vi "VISA_ReadAndSave_2CHparalelos.vi"() -> ()   [LabVIEW 2019]
uses:
  813f916b-c519-439e-9418-14bd48b6d342.vi
  <vilib>/Instr/_visa.llb/VISA Configure Serial Port (Instr).vi
  <vilib>/Analysis/Matrix/Comparison/Not Equal/Not Equal.vi
  <vilib>/Analysis/Matrix/Comparison/Not Equal/Not Equal - RM,RM.vi
panel:
  out "error file":errorcluster
  in  "file name":string
  out "Plot 1":dbl[](graph)
  out "Plot 0":dbl[](graph)
  out "Status Read":errorcluster
  out "Buffer Array":dbl[](array[numeric])
  out "Read Buffer":string
  out "Status Serial":errorcluster
  in  "Stop Read":bool
  in  "Start Read":bool
  in  "baud rate (9600)":u32=115200
  in  "data bits (8)":u8=8 min=5 max=8 step=1
  in  "VISA resource name":refnum<visa-resource-name>
  # "Controle de Salvamento"
  # "Log de Erros"
  # "Conversão Para Inteiro"
  # "Resultado da Leitura"
  # "Controle da porta Serial USB"
  # "Controle da Leitura"
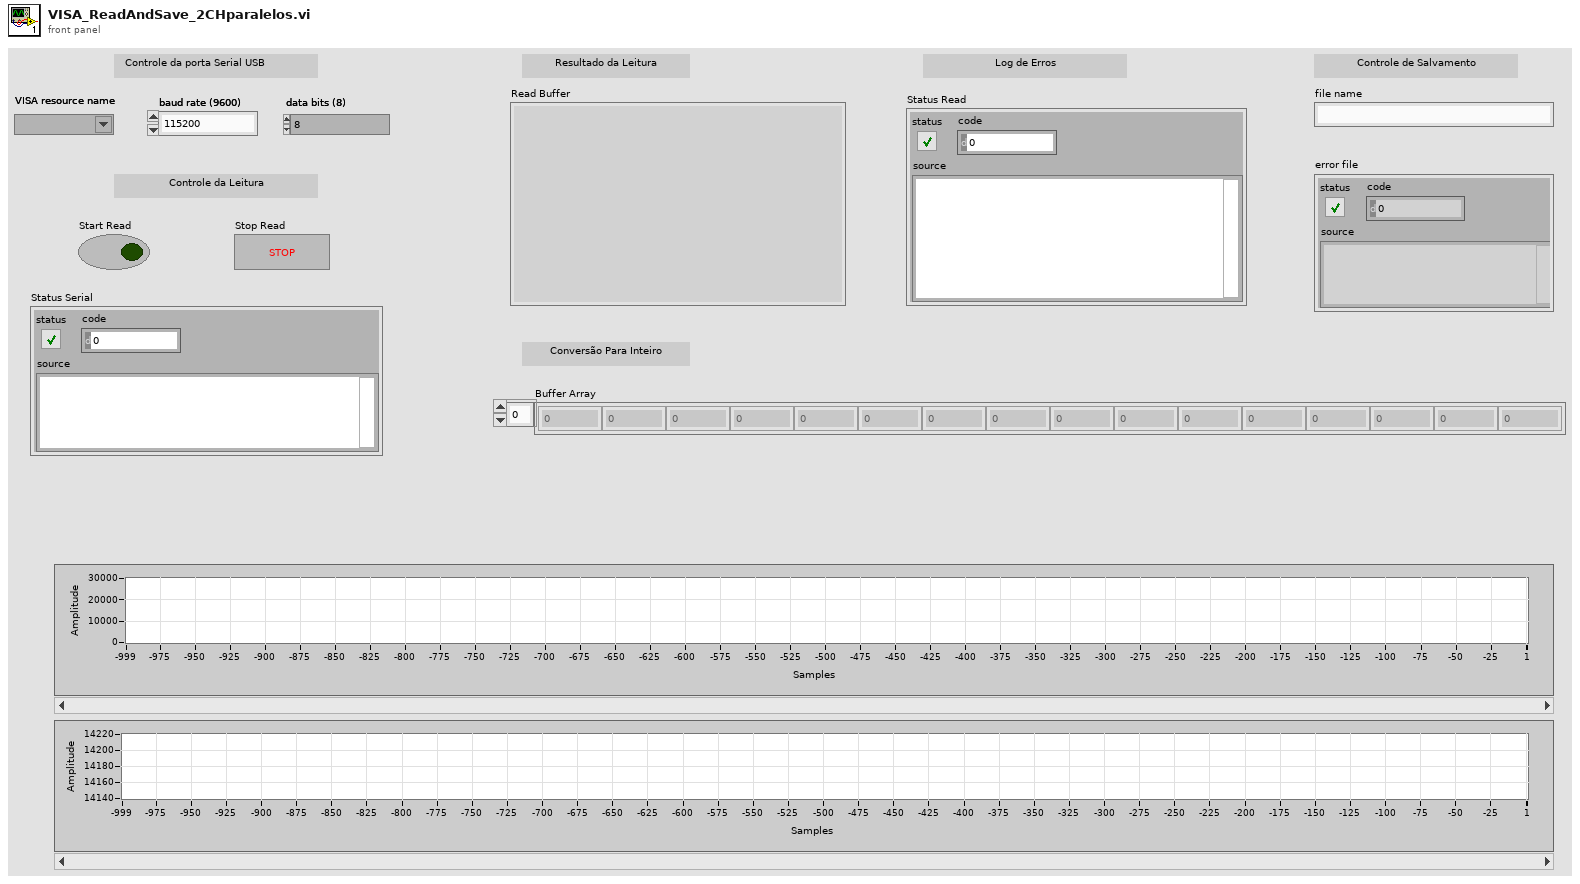
[diagram p1: front panel]
types:
  T1 = typedef "NI_Matrix.lvlib/RealMatrix.ctl" = dbl[][]
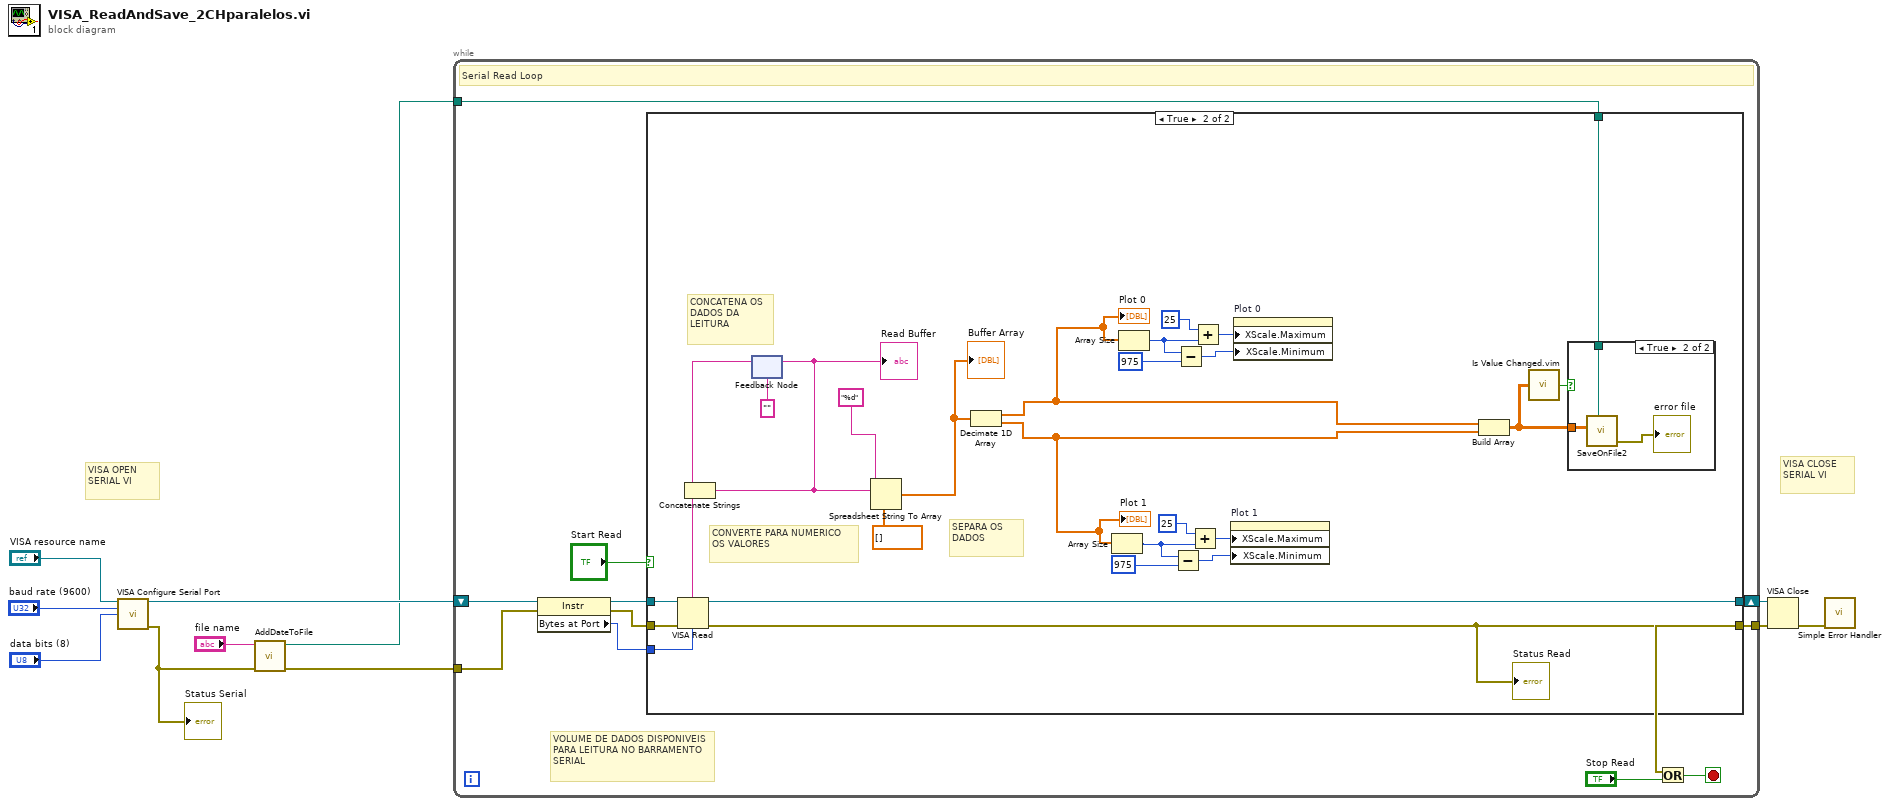
[diagram p0: block diagram]
diagram:
  # "VISA OPEN SERIAL VI"
  # "VISA CLOSE SERIAL VI"
  n1 = call-poly "VISA Configure Serial Port"("VISA resource name"="VISA resource name", "baud rate (9600)"="baud rate (9600)", "data bits (8)"="data bits (8)") -> ("VISA resource name out"=w9:refnum<visa-resource-name>, "error out"=w2:errorcluster)  [unwired: 11 in]
  "Status Serial" <- w2
  n2 = call "AddDateToFile.vi"("error in (no error)"=w2, "file name"="file name") -> ("error out"=w3:errorcluster, "new file path (Not A Path if cancelled)"=w1:path)  [unwired: 8 in]
  n3 = while {
    tunnel: w3 -> [w13]
    tunnel: [w20] -> w10
    shift-right: [w19] -> w8
    shift-left: w9 -> [w17]
    tunnel: w1 -> [w12]
    stop <- w18 stop-if-true
    # "VOLUME DE DADOS DISPONIVEIS PARA LEITURA NO BARRAMENTO SERIAL"
    # "Serial Read Loop"
    n4 = property class="Instr"(reference=w17, error in=w13) -> (reference out=w14:refnum<visa-resource-name>, error out=w15:errorcluster, "Bytes at Port"=w16:u32)
    n5 = case shown="True" "Start Read" {
      tunnel: [w23 w51] -> w20
      tunnel: [w24 w49] -> w19
      tunnel: w16 -> [_ w45]
      tunnel: w14 -> [w24 w44]
      tunnel: w15 -> [w23 w43]
      tunnel: w12 -> [_ w31]
      frame False {
        # "OS DADOS SÃO ACUMULADOS NO BUFFER ESPERANDO A PERMISSÃO PARA SER LIDOS"
      }
      frame True {
        # "SEPARA OS DADOS"
        # "CONVERTE PARA NUMERICO OS VALORES"
        # "CONCATENA OS DADOS DA LEITURA"
        n6 = VISA Read(VISA resource name=w44, byte count=w45, error in (no error)=w43) -> (VISA resource name out=w49:refnum<visa-resource-name>, read buffer=w40:string, error out=w51:errorcluster)  [unwired: 1 out]
        "Status Read" <- w51
        n7 = feedback #1("") -> (w46:string)
        n8 = Concatenate Strings(w46, w40) -> (w48:string)
        "Read Buffer" <- w48
        n9 = feedback-in #1(w48) -> ()
        n10 = Spreadsheet String To Array(format string="%d", spreadsheet string=w48, array type (2D Dbl)=dbl[] []) -> (array=w41:dbl[])  [unwired: 1 in]
        "Buffer Array" <- w41
        n11 = Decimate 1D Array(w41) -> (w32:dbl[], w25:dbl[])
        "Plot 0" <- w32
        "Plot 1" <- w25
        n12 = Array Size(array=w25) -> (size(s)=w27:i32)
        n13 = Array Size(array=w32) -> (size(s)=w35:i32)
        n14 = Subtract(x=w27, y=975) -> (x-y=w30:i32)
        n15 = Subtract(x=w35, y=975) -> (x-y=w36:i32)
        n16 = Add(x=25, y=w27) -> (x+y=w29:i32)
        n17 = Add(x=25, y=w35) -> (x+y=w34:i32)
        n18 = property on="Plot 1" class="WFGraph (strict)"("XScale.Maximum"=w29, "XScale.Minimum"=w30) -> ()  [unwired: 2 in, 2 out]
        n19 = property on="Plot 0" class="WFGraph (strict)"("XScale.Maximum"=w34, "XScale.Minimum"=w36) -> ()  [unwired: 2 in, 2 out]
        n20 = Build Array(w32, w25) -> (w39:T1)
        n21 = call "Is Value Changed.vim"("value"=w39) -> ("changed or first call?"=w38:bool)
        n22 = case shown="True" w38 {
          tunnel: w39 -> [_ w52]
          tunnel: w31 -> [_ w54]
          frame False {
          }
          frame True {
            n23 = call "SaveOnFile2.vi"("2D data"=w52, "file path (dialog if empty)"=w54) -> ("error file"=→"error file":errorcluster)  [unwired: 5 in]
          }
        }
      }
    }
    n24 = Or(x=w20, y="Stop Read") -> (x .or. y?=w18:bool)
  }
  n25 = VISA Close(VISA resource name=w8, error in (no error)=w10) -> (error out=w7:errorcluster)
  n26 = call <vilib>:"Simple Error Handler.vi"("error in (no error)"=w7) -> ()  [unwired: 4 in, 5 out]
